vi "Write CLI.vi"(10 "CLI":refnum<class "CLI.lvclass">, 11 "Wiresmith CLI Output in":refnum<class "Wiresmith CLI Output.lvclass">) -> (3 "Wiresmith CLI Output out":refnum<class "Wiresmith CLI Output.lvclass">)   [LabVIEW 2019, in "Wiresmith CLI Output.lvclass"]
uses:
  Wiresmith CLI Output.lvclass
  <vilib>/Wiresmith Technology/G CLI/CLI Class/CLI.lvclass
  Wiresmith CLI Output.lvclass/Wiresmith CLI Output.ctl
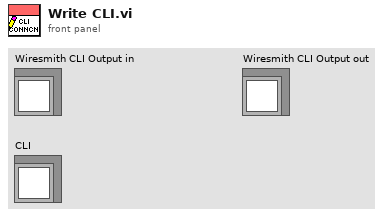
[diagram p1: front panel]
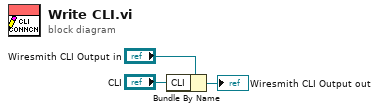
[diagram p0: block diagram]
diagram:
  n1 = Bundle By Name(cluster="Wiresmith CLI Output in", "CLI"="CLI") -> (→"Wiresmith CLI Output out":refnum<class "Wiresmith CLI Output.lvclass">)
